vi "Read RawData.vi"(8 "error in (no error)":errorcluster, 9 "WCM_max_value":bool, 10 "# of scans":i32, 11 "UV-VIS_AVANTES in":refnum<class "UV-VIS_AVANTES.lvclass">) -> (0 "error out":errorcluster, 1 "Channel II":sgl[][](array[numeric]), 2 "Channel I":sgl[][](array[numeric]), 3 "UV-VIS_AVANTES out":refnum<class "UV-VIS_AVANTES.lvclass">, 4 "WCM_values":sgl[](array[numeric]))   [LabVIEW 2015, in "UV-VIS_AVANTES.lvclass"]
uses:
  UV-VIS_AVANTES.lvclass
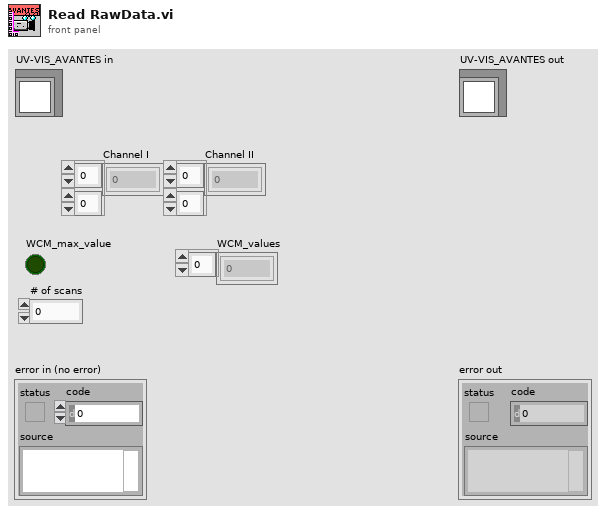
[diagram p1: front panel]
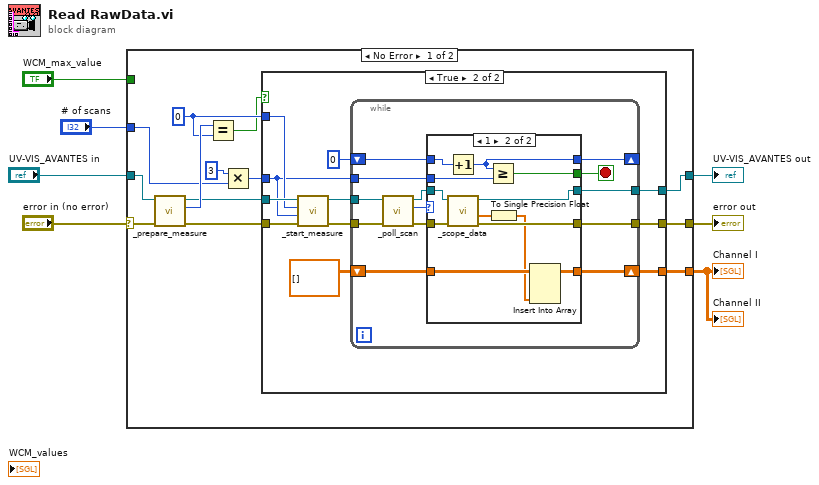
[diagram p0: block diagram]
diagram:
  n1 = case shown="No Error" "error in (no error)" {
    selector: "error in (no error)" -> [w19 w64]
    tunnel: [w11 w64] -> w6
    tunnel: [w12 w63] -> w5
    tunnel: "UV-VIS_AVANTES in" -> [w20 w63]
    tunnel: "# of scans" -> [w10 _]
    tunnel: "WCM_max_value" -> [_ _]
    tunnel: [w14 _] -> w1
    frame No Error {
      w15 = 0 ("y")
      n2 = call "_prepare_measure.vi"("error in (no error)"=w19, "UV-VIS_AVANTES in"=w20) -> ("error out"=w17:errorcluster, "return type"=w18:i32, "UV-VIS_AVANTES out"=w16:refnum<class "UV-VIS_AVANTES.lvclass">)  [unwired: 7 in]
      n3 = Equal?(x=w18, y=w15) -> (x = y?=w13:bool)
      n4 = Multiply(x=3, y=w10) -> (x*y=w8:i32)
      n5 = case shown="True" w13 {
        tunnel: w17 -> [w21 w33]
        tunnel: w16 -> [w22 w32]
        tunnel: w15 -> [_ w31]
        tunnel: [_ w29] -> w14
        tunnel: w8 -> [_ w27]
        tunnel: [w22 w24] -> w12
        tunnel: [w21 w23] -> w11
        frame False {
        }
        frame True {
          n6 = call "_start_measure.vi"("error in (no error)"=w33, "a_Nmsr"=w27, "a_hWnd"=w31, "UV-VIS_AVANTES in"=w32) -> ("error out"=w25:errorcluster, "UV-VIS_AVANTES out"=w26:refnum<class "UV-VIS_AVANTES.lvclass">)  [unwired: 6 in]
          n7 = while {
            shift-right: [w45] -> w29
            shift-left: sgl[][] [] ("32bit integer") -> [w44]
            shift-right: [w43] -> _
            shift-left: 0 -> [w42]
            tunnel: w27 -> [w41]
            tunnel: w26 -> [w39]
            tunnel: w25 -> [w38]
            tunnel: [w35] -> w24
            tunnel: [w34] -> w23
            stop <- w40 stop-if-true
            n8 = call "_poll_scan.vi"("error in (no error)"=w38, "UV-VIS_AVANTES in"=w39) -> ("error out"=w36:errorcluster, "return"=w46:i32, "UV-VIS_AVANTES out"=w37:refnum<class "UV-VIS_AVANTES.lvclass">)  [unwired: 7 in]
            n9 = case shown="1" w46 {
              tunnel: [w50 w57] -> w45
              tunnel: w44 -> [w50 w58]
              tunnel: [w49 w61] -> w43
              tunnel: w42 -> [w49 w62]
              tunnel: w41 -> [_ w60]
              tunnel: [_ w59] -> w40
              tunnel: w37 -> [w48 w56]
              tunnel: w36 -> [w47 w55]
              tunnel: [w48 w54] -> w35
              tunnel: [w47 w53] -> w34
              frame 0, Default {
              }
              frame 1 {
                n10 = Increment(x=w62) -> (x+1=w61:i32)
                n11 = call "_scope_data.vi"("error in (no error)"=w55, "UV-VIS_AVANTES in"=w56) -> ("error out"=w53:errorcluster, "a_pSpectrum"=w52:dbl[], "UV-VIS_AVANTES out"=w54:refnum<class "UV-VIS_AVANTES.lvclass">)  [unwired: 6 in, 1 out]
                n12 = Greater Or Equal?(x=w61, y=w60) -> (x >= y?=w59:bool)
                n13 = To Single Precision Float(number=w52) -> (single precision float=w51:sgl[])
                n14 = Insert Into Array(array=w58, new element=w51) -> (w57:sgl[][])  [unwired: 2 in]
              }
            }
          }
        }
      }
    }
    frame Error {
    }
  }
  "error out" <- w6
  "UV-VIS_AVANTES out" <- w5
  "Channel II" <- w1
  "Channel I" <- w1
